vi "Set Input Power Name.vi"(8 "error in (no error)":errorcluster, 10 "Input Power Name":string, 11 "Test Group In":refnum<data-value>) -> (0 "error out":errorcluster, 3 "Test Group Out":refnum<data-value>)   [LabVIEW 2016, in "Test Group Manager.lvlib" / "Test Group.lvclass"]
uses:
  Test Group.lvclass
  Test Group.lvclass/Test Group.ctl
  Read Test Group Data.vi
  Write Test Group Data.vi
  Write Input Power Initialized.vi
  Read Input Power Initialized.vi
  <vilib>/Utility/error.llb/Error Cluster From Error Code.vi
  <vilib>/ErrorRing/Error Ring.xnode
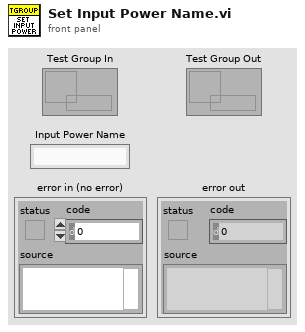
[diagram p1: front panel]
types:
  T1 = cluster{"DPD LUT Name":string, "Input Power":string}
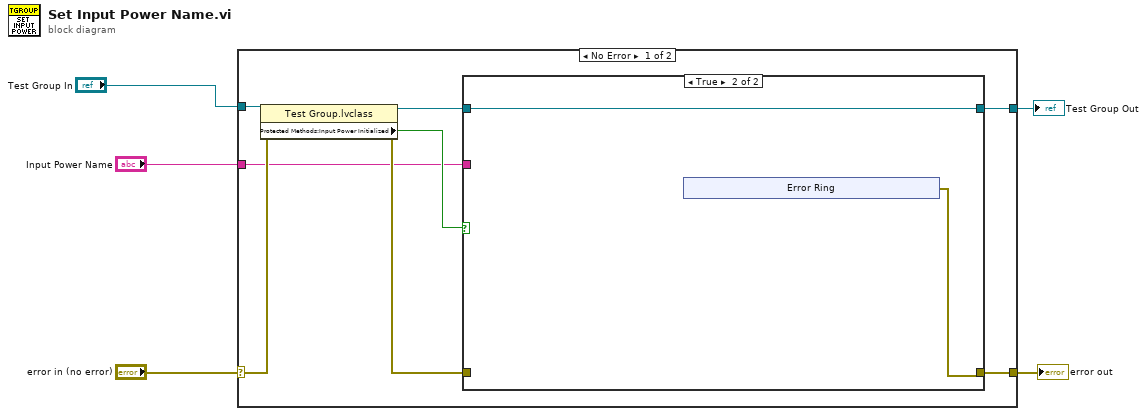
[diagram p0: block diagram]
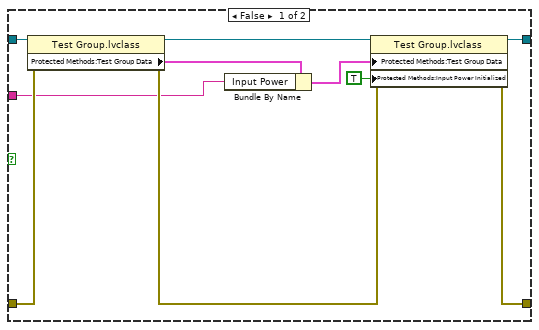
[diagram p2: hidden frame]
diagram:
  n1 = case shown="No Error" "error in (no error)" {
    selector: "error in (no error)" -> [w13 w32]
    tunnel: [w12 w32] -> w4
    tunnel: "Input Power Name" -> [w8 _]
    tunnel: "Test Group In" -> [w7 w31]
    tunnel: [w6 w31] -> w1
    frame No Error {
      n2 = property class="Test Group.lvclass"(reference=w7, error in=w13) -> (reference out=w9:refnum<data-value>, error out=w11:errorcluster, "Protected Methods:Input Power Initialized"=w10:bool)
      n3 = case shown="True" w10 {
        tunnel: [w22 w25] -> w12
        tunnel: w11 -> [w23 _]
        tunnel: [w21 w24] -> w6
        tunnel: w9 -> [w19 w24]
        tunnel: w8 -> [w15 _]
        frame False {
          n4 = property class="Test Group.lvclass"(reference=w19, error in=w23) -> (reference out=w18:refnum<data-value>, error out=w20:errorcluster, "Protected Methods:Test Group Data"=w17:T1)
          n5 = Bundle By Name(cluster=w17, "Input Power"=w15) -> (w16:T1)
          n6 = property class="Test Group.lvclass"(reference=w18, error in=w20, "Protected Methods:Test Group Data"=w16, "Protected Methods:Input Power Initialized"=TRUE ("DPD Initialized")) -> (reference out=w21:refnum<data-value>, error out=w22:errorcluster)
        }
        frame True {
          n7 = xnode "Error Ring"() -> ("error out"=w25:errorcluster)
        }
      }
    }
    frame Error {
    }
  }
  "error out" <- w4
  "Test Group Out" <- w1
